vi "Dialog - Settings.vi"(7 "Data (in)":T1) -> (8 "Data (out)":T1)   [LabVIEW 2020]
uses:
  TypeDefs/Data.ctl
panel:
  in  "Cancel Button":bool
  in  "Hide Zero Values?":bool
  in  "Align Columns?":bool
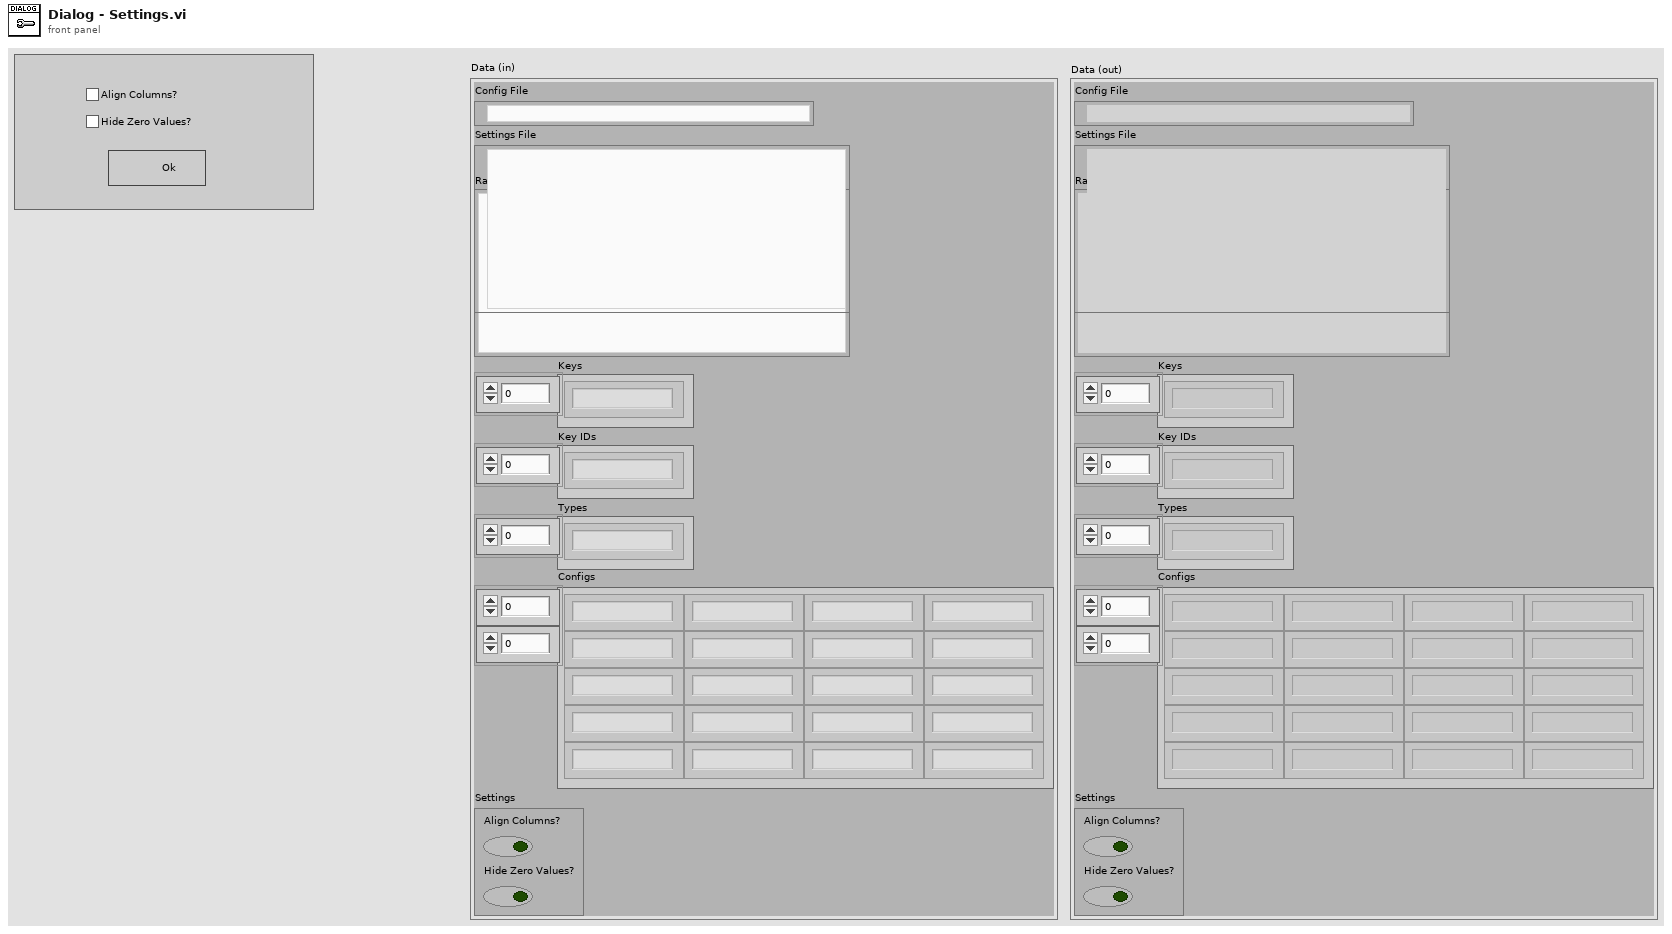
[diagram p1: front panel]
types:
  T1 = typedef "Data.ctl" = cluster{"Config File":path, "Settings File":path, "Raw Config Data":string, "Keys":string[], "Key IDs":string[], "Types":string[], "Configs":string[][], "Settings":cluster{"Align Columns?":bool, "Hide Zero Values?":bool}}
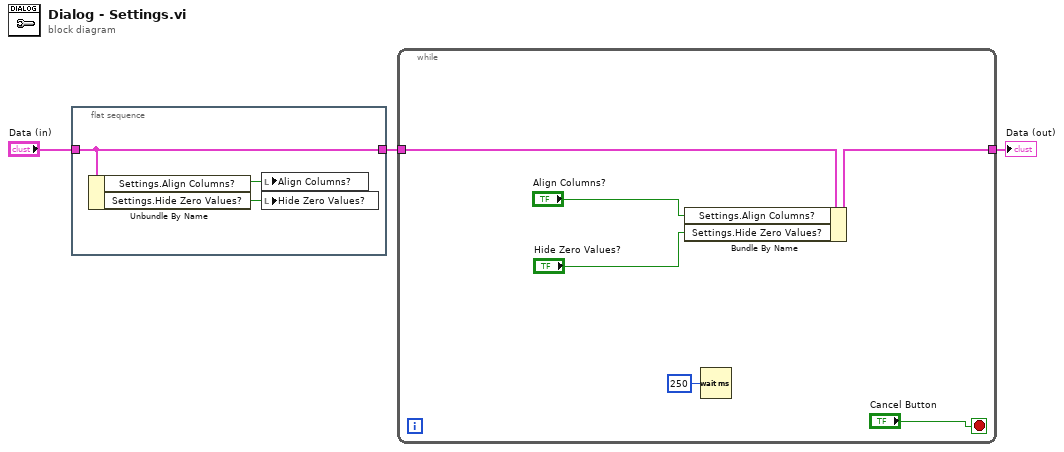
[diagram p0: block diagram]
diagram:
  n1 = flat-sequence {
    tunnel: "Data (in)" -> [w4]
    tunnel: [w4] -> w1
    frame #0 {
      n2 = Unbundle By Name(w4) -> ("Settings.Align Columns?"=w6:bool, "Settings.Hide Zero Values?"=w5:bool)
      n3 = local write "Align Columns?"(w6) -> ()
      n4 = local write "Hide Zero Values?"(w5) -> ()
    }
  }
  n5 = while {
    tunnel: w1 -> [w10]
    tunnel: [w9] -> w3
    stop <- "Cancel Button" stop-if-true
    n6 = Bundle By Name(cluster=w10, "Settings.Align Columns?"="Align Columns?", "Settings.Hide Zero Values?"="Hide Zero Values?") -> (w9:T1)
    n7 = Wait (ms)(milliseconds to wait=u32 250) -> ()  [unwired: 1 out]
  }
  "Data (out)" <- w3
